vi "Custom Types in Meta Data.vi"() -> ()   [LabVIEW 2020, in "NI_VIAnCFGDataStructure.lvlib" / "Tree.lvclass"]
uses:
  <vilib>/addons/analyzer/VIAnCFGDataStructure/Tree Manager/Tree.lvclass
  <vilib>/addons/analyzer/VIAnCFGDataStructure/Data Types/Error Cluster/Error Cluster.lvclass
  e:/builds/penguin/labview/branches/2020/dev/dist/vi.lib/addons/analyzer/VIAnCFGDataStructure/Tree Data/Tree Data.lvclass
  <vilib>/addons/analyzer/VIAnCFGDataStructure/Data Types/Bool/Bool.lvclass/Bool.ctl
  <vilib>/addons/analyzer/VIAnCFGDataStructure/Data Types/Bool/To Bool Tree Data.vi
  <vilib>/addons/analyzer/VIAnCFGDataStructure/Data Types/Bool/From Bool Tree Data.vi
  <vilib>/Utility/error.llb/Clear Errors.vi
  <vilib>/addons/analyzer/VIAnCFGDataStructure/Data Types/Int/Int.lvclass
  <vilib>/addons/analyzer/VIAnCFGDataStructure/Data Types/Float/Flt.lvclass
  <vilib>/addons/analyzer/VIAnCFGDataStructure/Data Types/Bool/Bool.lvclass
  <vilib>/addons/analyzer/VIAnCFGDataStructure/Data Types/String/String.lvclass
  <vilib>/addons/analyzer/VIAnCFGDataStructure/Data Types/Path/Path.lvclass
  <vilib>/addons/analyzer/VIAnCFGDataStructure/Data Types/Int Array/1D Int.lvclass
  <vilib>/addons/analyzer/VIAnCFGDataStructure/Data Types/Flt Array/1D Flt.lvclass
  <vilib>/addons/analyzer/VIAnCFGDataStructure/Data Types/Bool Array/1D Bool.lvclass
  <vilib>/addons/analyzer/VIAnCFGDataStructure/Data Types/String Array/1D String.lvclass
  <vilib>/addons/analyzer/VIAnCFGDataStructure/Data Types/Path Array/1D Path.lvclass
  <vilib>/addons/analyzer/VIAnCFGDataStructure/Data Types/2D Int/2D Int.lvclass
  <vilib>/addons/analyzer/VIAnCFGDataStructure/Data Types/2D Flt/2D Flt.lvclass
  <vilib>/addons/analyzer/VIAnCFGDataStructure/Data Types/2D Bool/2D Bool.lvclass
  <vilib>/addons/analyzer/VIAnCFGDataStructure/Data Types/2D String/2D String.lvclass
  <vilib>/addons/analyzer/VIAnCFGDataStructure/Data Types/2D Path/2D Path.lvclass
  <vilib>/Utility/Data Type/Get Type Information.vi
  <vilib>/Utility/error.llb/Error Cluster From Error Code.vi
  <vilib>/Utility/Data Type/Get Array Information.vi
  <vilib>/addons/analyzer/VIAnCFGDataStructure/Tree Manager/API/Set Attribute Tree Data.vi
  <vilib>/addons/analyzer/VIAnCFGDataStructure/Tree Manager/API/Get Attribute Tree Data.vi
  <vilib>/addons/analyzer/VIAnCFGDataStructure/Tree Data/Tree Data.lvclass
  e:/builds/penguin/labview/branches/2020/dev/dist/vi.lib/addons/analyzer/VIAnCFGDataStructure/Data Types/Bool/Bool.lvclass
  <vilib>/addons/analyzer/VIAnCFGDataStructure/Data Types/Int/From Integer Tree Data.vi
panel:
  in  "Tab Control":T1(tab)
  in  "Input Error Cluster":errorcluster={"status"=TRUE, "code"=123, "source"="Some description."}
  out "Extracted From Meta Data":errorcluster={"status"=TRUE, "code"=123, "source"="Some description."}
  out "Extracted From Error Cluster TD Type":errorcluster={"status"=TRUE, "code"=123, "source"="Some description."}
  out "Error Status":bool=TRUE
  in  "Tree":string(tree)
  out "XML String":string="<Parent>\n\n<Child>\n<Attr Name=\"Custom Error Type\" Type=\"Bool\" MetaData=\"<Cluster>\r\n<Name>Input Error Cluster</Name>\r\n<NumElts>3</NumElts>\r\n<Boolean>\r\n<Name>status</Name>\r\n<Val>1</Val>\r\n</Boolean>\r\n<I32>\r\n<Name>code</Name>\r\n<Val>123</Val>\r\n</I32>\r\n<String>\r\n<Name>source</Name>\r\n<Val>Some description.</Val>\r\n</String>\r\n</Cluster>\r\n\">TRUE</Attr>\r\n<Attr Name=\"Error Cluster Type\" Type=\"Error Cluster\" >TRUE, 123</Attr>\n\n</Child>\n</Parent>"
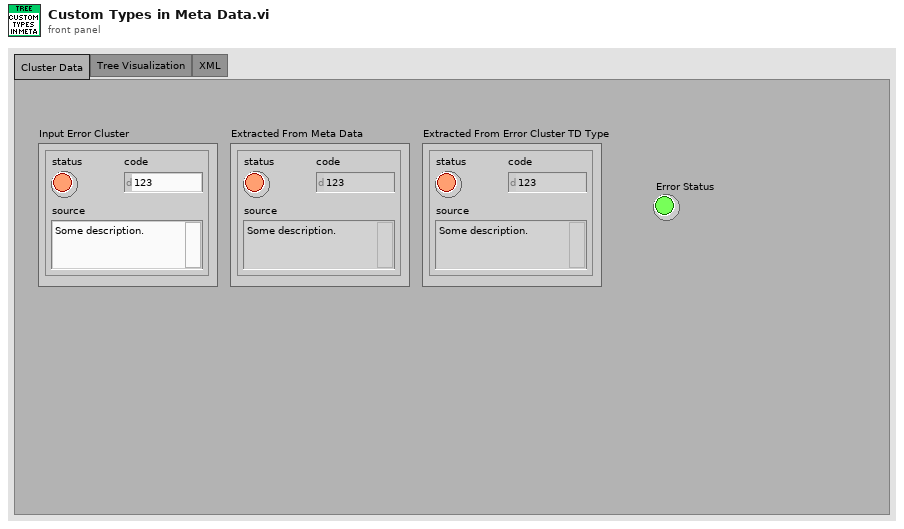
[diagram p1: front panel]
types:
  T1 = enum32{"Cluster Data", "Tree Visualization", "XML"}
  T2 = typedef "NI_VIAnCFGDataStructure.lvlib/Tree.lvclass/Session Handle.ctl" = refnum<data-value>
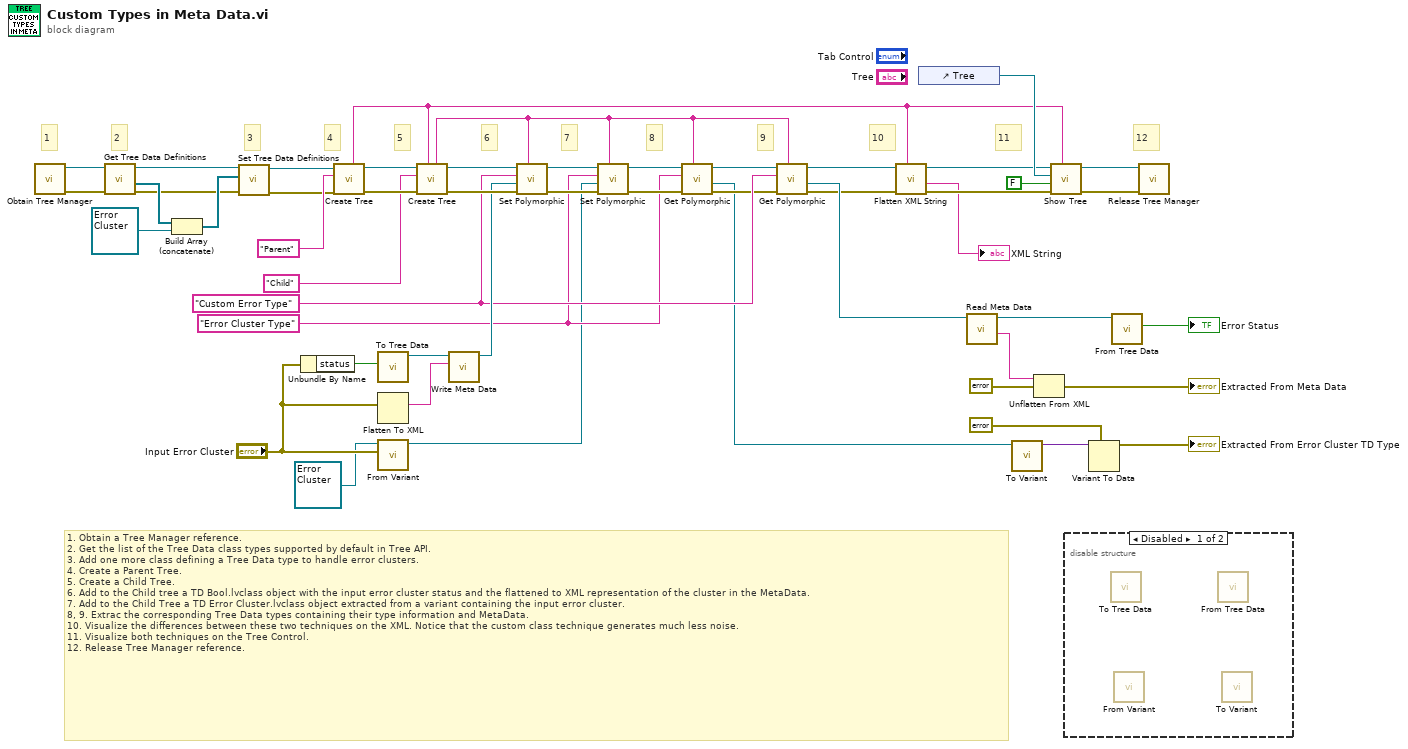
[diagram p0: block diagram]
diagram:
  w24 = "Error Cluster Type" ("Name")
  w39 = "Custom Error Type" ("Name")
  # "1. Obtain a Tree Manager reference.\n2. Get the list of the Tree Data class types supported by default in Tree API.\n3. Add one more class defining a Tree Data type to handle error clusters.\n4. Create a Parent Tree.\n5. Create a Child Tree.\n6. Add to the Child tree a TD Bool.lvclass object with the input error cluster status and the flattened to XML representation of the cluster in the MetaData.\n7. Add to the Child Tree a TD Error Cluster.lvclass object extracted from a variant containing the input error cluster.\n8, 9. Extrac the corresponding Tree Data types containing their type information and MetaData.\n10. Visualize the differences between these two techniques on the XML. Notice that the custom class technique generates much less noise.\n11. Visualize both techniques on the Tree Control.\n12. Release Tree Manager reference."
  # "12"
  # "11"
  # "10"
  # "9"
  # "8"
  # "7"
  # "6"
  # "5"
  # "4"
  # "3"
  # "2"
  # "1"
  n1 = call <vilib>:"Obtain Tree Manager.vi"() -> ("Error Out"=w16:errorcluster, "Tree"=w17:T2)  [unwired: 10 in]
  n2 = call <vilib>:"Get Tree Data Definitions.vi"("Error In"=w16, "Tree Manager"=w17) -> ("Error Out"=w11:errorcluster, "Tree Data Defs"=w14:refnum<class "Tree Data.lvclass">[], "Tree Manager"=w15:T2)  [unwired: 7 in]
  n3 = Build Array (concatenate)(w14, refnum<class "Error Cluster.lvclass"> refnum ("TD Error Cluster.lvclass")) -> (w12:refnum<class "Tree Data.lvclass">[])
  n4 = call <vilib>:"Set Tree Data Definitions.vi"("Error In"=w11, "Tree Data Defs"=w12, "Tree Manager"=w15) -> ("Error Out"=w10:errorcluster, "Tree Manager"=w9:T2)  [unwired: 7 in]
  n5 = Unbundle By Name("Input Error Cluster") -> ("status"=w36:bool)
  n6 = call <vilib>:"Create Tree.vi"("Error In"=w10, "Name"="Parent", "Tree Manager"=w9) -> ("Error Out"=w50:errorcluster, "Tree Manager"=w51:T2, "Unique ID"=w7:string)  [unwired: 6 in]
  n7 = call-poly <vilib>:"To Tree Data.vi"("Boolean"=w36) -> ("Bool Tree Data"=w41:refnum<class "Bool.lvclass">)  [unwired: 10 in]
  n8 = Flatten To XML(6:"Input Error Cluster") -> (2:w35:string)
  n9 = call <vilib>:"From Variant.vi"("Variant"="Input Error Cluster", "Tree Data Type"=refnum<class "Error Cluster.lvclass"> refnum ("TD Error Cluster.lvclass")) -> ("Tree Data Out"=w19:refnum<class "Tree Data.lvclass">)  [unwired: 8 in, 1 out]
  n10 = call <vilib>:"Create Tree.vi"("Parent ID (empty)"=w7, "Error In"=w50, "Name"="Child", "Tree Manager"=w51) -> ("Error Out"=w45:errorcluster, "Tree Manager"=w46:T2, "Unique ID"=w27:string)  [unwired: 5 in]
  n11 = call <vilib>:"Write Meta Data.vi"("Meta Data"=w35, "Tree Data In"=w41) -> ("Tree Data Out"=w44:refnum<class "Bool.lvclass">)  [unwired: 9 in]
  n12 = call-poly <vilib>:"Set Polymorphic.vi"("Tree ID"=w27, "Error In"=w45, "Attribute Value"=w44, "Attribute Name"=w39, "Tree Manager"=w46) -> ("Error Out"=w30:errorcluster, "Tree Manager"=w31:T2)  [unwired: 4 in, 1 out]
  n13 = call-poly <vilib>:"Set Polymorphic.vi"("Tree ID"=w27, "Error In"=w30, "Attribute Value"=w19, "Attribute Name"=w24, "Tree Manager"=w31) -> ("Error Out"=w28:errorcluster, "Tree Manager"=w29:T2)  [unwired: 4 in, 1 out]
  n14 = call-poly <vilib>:"Get Polymorphic.vi"("Tree ID"=w27, "Error In"=w28, "Attribute Name"=w24, "Tree Manager"=w29) -> ("Error Out"=w25:errorcluster, "Attribute Value"=w23:refnum<class "Tree Data.lvclass">, "Tree Manager"=w26:T2)  [unwired: 4 in, 1 out]
  n15 = call-poly <vilib>:"Get Polymorphic.vi"("Tree ID"=w27, "Error In"=w25, "Attribute Name"=w39, "Tree Manager"=w26) -> ("Error Out"=w6:errorcluster, "Attribute Value"=w38:refnum<class "Tree Data.lvclass">, "Tree Manager"=w8:T2)  [unwired: 4 in, 1 out]
  n16 = call <vilib>:"Flatten XML String.vi"("Root ID"=w7, "Error In"=w6, "Tree"=w8) -> ("Error Out"=w4:errorcluster, "XML String"=→"XML String":string, "Tree"=w5:T2)  [unwired: 6 in]
  n17 = control-ref of="Tree"() -> (w47:refnum<vi>)
  n18 = call <vilib>:"Read Meta Data.vi"("Tree Data In"=w38) -> ("Meta Data"=w32:string, "Tree Data Out"=w37:refnum<class "Tree Data.lvclass">)  [unwired: 9 in]
  n19 = call <vilib>:"To Variant.vi"("Tree Data"=w23) -> ("Variant"=w22:variant)  [unwired: 9 in, 1 out]
  n20 = Unflatten From XML(xml string=w32, type=errorcluster {"status"=FALSE, "code"=0, "source"=""} ("error in (no error)")) -> (value=→"Extracted From Meta Data":errorcluster)  [unwired: 1 in, 1 out]
  n21 = call <vilib>:"Show Tree.vi"("Root ID"=w7, "Error In"=w4, "Show IDs (False)"=FALSE ("Show IDs (True)"), "Tree Ref"=w47, "Tree"=w5) -> ("Error Out"=w42:errorcluster, "Tree"=w43:T2)  [unwired: 5 in]
  n22 = disable-structure shown="Disabled" {
    frame Disabled {
      n23 = call-poly <vilib>:"To Tree Data.vi"() -> ()  [unwired: 11 in, 1 out]
      n24 = call <vilib>:"From Variant.vi"() -> ()  [unwired: 10 in, 2 out]
      n25 = call-poly <vilib>:"From Tree Data.vi"() -> ()  [unwired: 11 in, 1 out]
      n26 = call <vilib>:"To Variant.vi"() -> ()  [unwired: 10 in, 2 out]
    }
    frame Enabled {
    }
  }
  n27 = Variant To Data(type=errorcluster {"status"=FALSE, "code"=0, "source"=""} ("error in (no error)"), Variant=w22) -> (data=→"Extracted From Error Cluster TD Type":errorcluster)  [unwired: 1 in, 1 out]
  n28 = call-poly <vilib>:"From Tree Data.vi"("Tree Data"=w37) -> ("Boolean"=→"Error Status":bool)  [unwired: 10 in]
  n29 = call <vilib>:"Release Tree Manager.vi"("Error In"=w42, "Tree"=w43) -> ()  [unwired: 9 in, 1 out]
